vi "Untitled 1 (SubVI).vi"   [LabVIEW 2015]
uses:
  Control Packet Type.ctl
  Control Packet - Basic.ctl
types:
  T1 = typedef "Control Packet - Basic.ctl" = cluster{"Boolean":bool}
  T2 = typedef "Control Packet Type.ctl" = enum8{"Basic"}
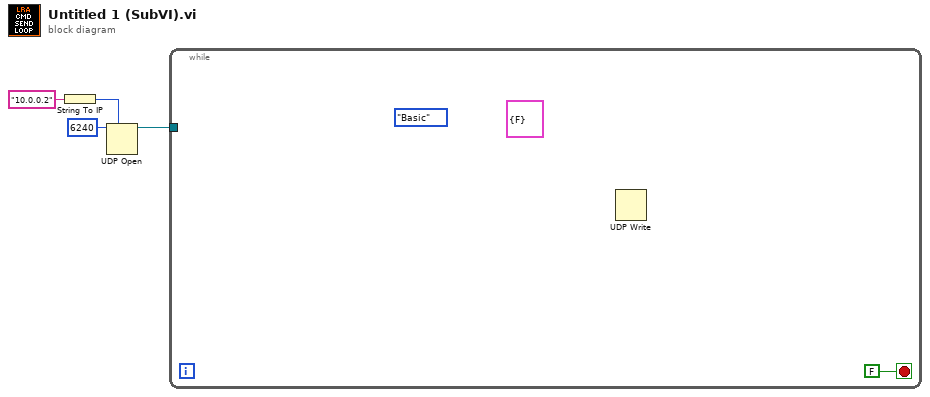
[diagram p0: block diagram]
diagram:
  n1 = String To IP(1:"10.0.0.2" ("name")) -> (0:w2:u32)
  n2 = UDP Open(7:w2, 11:u16 6240 ("port")) -> (port=w4:refnum<k16>)  [unwired: 3 in, 2 out]
  n3 = while {
    tunnel: w4 -> [_]
    stop <- FALSE stop-if-true
    (unwired) T1 {"Boolean"=FALSE}
    (unwired) Control_Packet_Type."Basic" ("Enum")
    n4 = UDP Write() -> ()  [unwired: 6 in, 2 out]
  }
